vi "ACQ task run.vi"(8 "error in (no error)":errorcluster, 11 "Tasks ref in":T1) -> (0 "error out":errorcluster, 3 "Tasks ref out":T1)   [LabVIEW 2013]
doc: "Use this template to build a VI to use as a subVI."
uses:
  Kontrolki/KartaDAQ/ACQ all read tasks.ctl
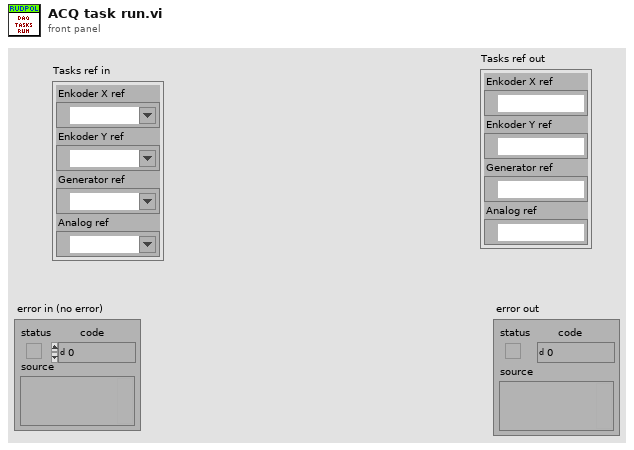
[diagram p1: front panel]
types:
  T1 = typedef "ACQ all read tasks.ctl" = cluster{"Enkoder X ref":refnum<k21>, "Enkoder Y ref":refnum<k21>, "Generator ref":refnum<k21>, "Analog ref":refnum<k21>}
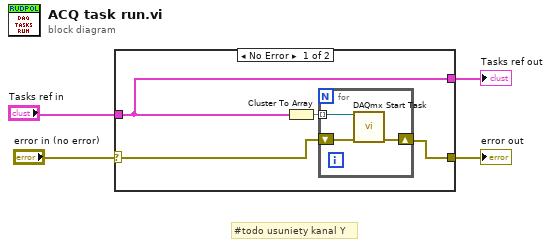
[diagram p0: block diagram]
diagram:
  # "#todo usuniety kanal Y"
  n1 = case shown="No Error" "error in (no error)" {
    selector: "error in (no error)" -> [w7 w13]
    tunnel: [w6 w13] -> w3
    tunnel: "Tasks ref in" -> [w5 w12]
    tunnel: [w5 w12] -> w1
    frame No Error {
      n2 = Cluster To Array(cluster=w5) -> (array=w8:refnum<k21>[])
      n3 = for {
        tunnel: w8 -> [w11] mode=indexing
        shift-right: [w9] -> w6
        shift-left: w7 -> [w10]
        n4 = call <vilib>:"DAQmx Start Task.vi"("task/channels in"=w11, "error in"=w10) -> ("error out"=w9:errorcluster)  [unwired: 12 in, 1 out]
      }
    }
    frame Error {
    }
  }
  "error out" <- w3
  "Tasks ref out" <- w1
